vi "Kick.vi"(8 "error in (no error)":errorcluster, 11 "Watchdog":refnum<data-value>) -> (0 "error out":errorcluster, 3 "Watchdog":refnum<data-value>)   [LabVIEW 2017, in "Watchdog.lvclass"]
doc: "Kick the watchdog (reset the internal timer)."
uses:
  <vilib>/NI/Software Watchdog/Watchdog/Watchdog.lvclass
  <vilib>/NI/Software Watchdog/Watchdog/Watchdog.lvclass/Watchdog.ctl
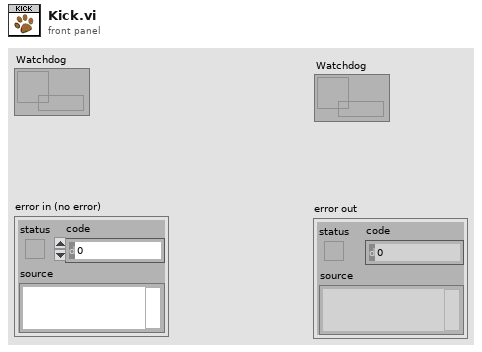
[diagram p1: front panel]
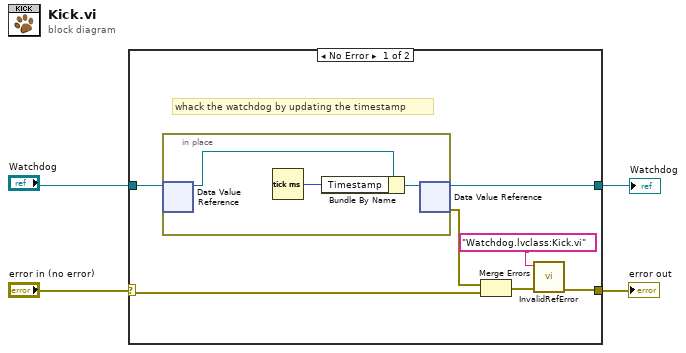
[diagram p0: block diagram]
diagram:
  n1 = case shown="No Error" "error in (no error)" {
    selector: "error in (no error)" -> [w5 w16]
    tunnel: [w9 w16] -> w3
    tunnel: "Watchdog" -> [w11 w15]
    tunnel: [w10 w15] -> w2
    frame No Error {
      # "whack the watchdog by updating the timestamp"
      n2 = in-place {
        n3 = in-place-dvr #1(w11) -> (w14:refnum<class "Watchdog.lvclass">)  [unwired: 1 out]
        n4 = Tick Count (ms)() -> (millisecond timer value=w12:u32)
        n5 = Bundle By Name(cluster=w14, "Timestamp"=w12) -> (w13:refnum<class "Watchdog.lvclass">)
        n6 = in-place-dvr #1(w13) -> (w10:refnum<data-value>, w6:errorcluster)
      }
      n7 = Merge Errors(w6, w5) -> (w7:errorcluster)
      n8 = call <vilib>:"InvalidRefError.vi"("error in (no error)"=w7, "VI Name"="Watchdog.lvclass:Kick.vi") -> ("error out"=w9:errorcluster)  [unwired: 9 in]
    }
    frame Error {
    }
  }
  "error out" <- w3
  "Watchdog" <- w2
